vi "Get HWnd From VI Ref.vi"(8 "error in (no error)":errorcluster, 10 "Remote Application?":bool, 11 "VI reference (calling VI)":refnum<vi>) -> (0 "error out":errorcluster, 3 "HWnd Out":u32)   [LabVIEW 2011]
doc: "This Vi will return the <B>HWnd Out</B> for a VI reference given by <B>VI reference (calling VI)</B>. If no reference is provided, this VI will use the calling VI reference and then close that reference after the HWnd has be read."
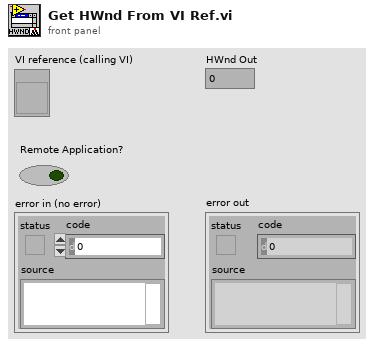
[diagram p1: front panel]
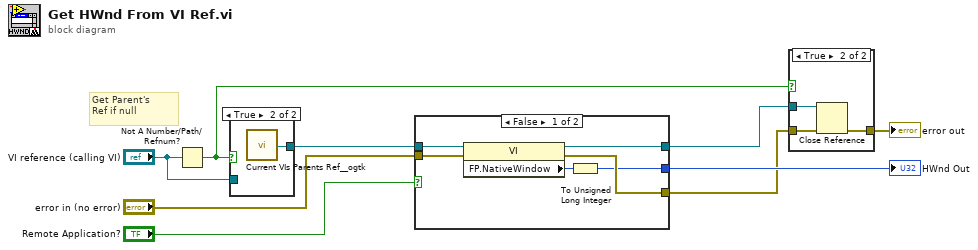
[diagram p0: block diagram]
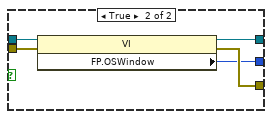
[diagram p2: hidden frame]
diagram:
  # "Get Parent's\nRef if null"
  n1 = Not A Number/Path/Refnum?(number/path/refnum="VI reference (calling VI)") -> (NaN/Path/Refnum?=w5:bool)
  n2 = case shown="True" w5 {
    tunnel: [w10 w11] -> w8
    tunnel: "VI reference (calling VI)" -> [w10 _]
    frame False {
    }
    frame True {
      n3 = call <userlib>:"Current VIs Parents Ref__ogtk.vi"() -> ("Calling VI's Reference"=w11:refnum<vi>)  [unwired: 2 in]
    }
  }
  n4 = case shown="False" "Remote Application?" {
    tunnel: w8 -> [w17 w22]
    tunnel: "error in (no error)" -> [w16 w21]
    tunnel: [w15 w19] -> w3
    tunnel: [w12 w18] -> w7
    tunnel: [w13 w20] -> w4
    frame False {
      n5 = property class="VI"(reference=w17, error in=w16) -> (reference out=w13:refnum<vi>, error out=w15:errorcluster, "FP.NativeWindow"=w14:u64)
      n6 = To Unsigned Long Integer(number=w14) -> (unsigned 32bit integer=w12:u32)
    }
    frame True {
      n7 = property class="VI"(reference=w22, error in=w21) -> (reference out=w20:refnum<vi>, error out=w19:errorcluster, "FP.OSWindow"=w18:i32)
    }
  }
  "HWnd Out" <- w7
  n8 = case shown="True" w5 {
    tunnel: w4 -> [_ w26]
    tunnel: w3 -> [w23 w25]
    tunnel: [w23 w24] -> w2
    frame False {
    }
    frame True {
      n9 = Close Reference(reference=w26, error in (no error)=w25) -> (error out=w24:errorcluster)
    }
  }
  "error out" <- w2
